vi "ArrayAverage.vi"() -> ()   [LabVIEW 2018]
panel:
  out "Array Average":dbl
  in  "Input Array":dbl[](array[numeric])
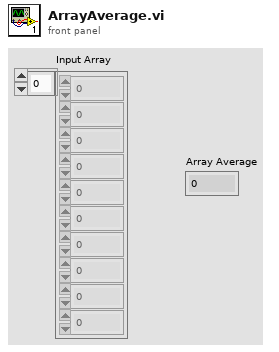
[diagram p1: front panel]
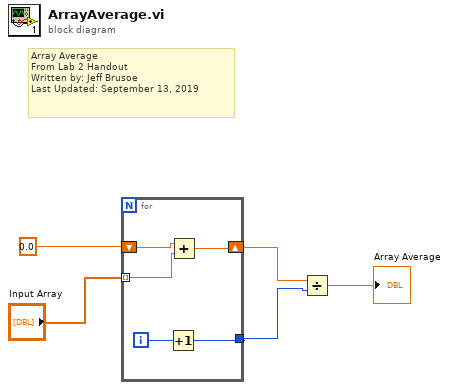
[diagram p0: block diagram]
diagram:
  # "Array Average\nFrom Lab 2 Handout\nWritten by: Jeff Brusoe\nLast Updated: September 13, 2019"
  n1 = for {
    tunnel: "Input Array" -> [w9] mode=indexing
    shift-right: [w8] -> w2
    shift-left: 0.0 -> [w10]
    tunnel: [w6] -> w1
    i -> [w7]
    n2 = Increment(x=w7) -> (x+1=w6:i32)
    n3 = Add(x=w10, y=w9) -> (x+y=w8:dbl)
  }
  n4 = Divide(x=w2, y=w1) -> (x/y=→"Array Average":dbl)
